vi "HRM-Stage4-init_main.vi"() -> (0 "error out":errorcluster, 3 "Init cluster":T1)   [LabVIEW 2020]
uses:
  HRM-Stage4-init_cluster.ctl
  HRM-Stage4-User_events.ctl
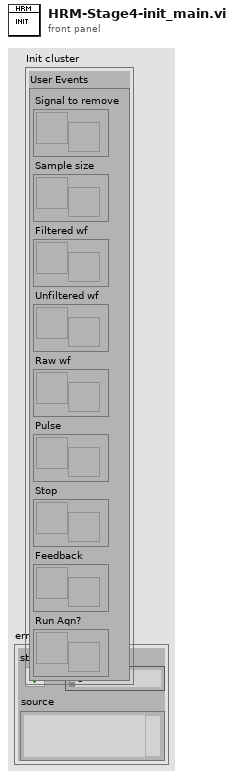
[diagram p1: front panel]
types:
  T1 = typedef "HRM-Stage4-init_cluster.ctl" = cluster{"User Events":T2}
  T2 = typedef "HRM-Stage4-User_events.ctl" = cluster{"Signal to remove":refnum<user-event>, "Sample size":refnum<user-event>, "Filtered wf":refnum<user-event>, "Unfiltered wf":refnum<user-event>, "Raw wf":refnum<user-event>, "Pulse":refnum<user-event>, "Stop":refnum<user-event>, "Feedback":refnum<user-event>, "Run Aqn?":refnum<user-event>}
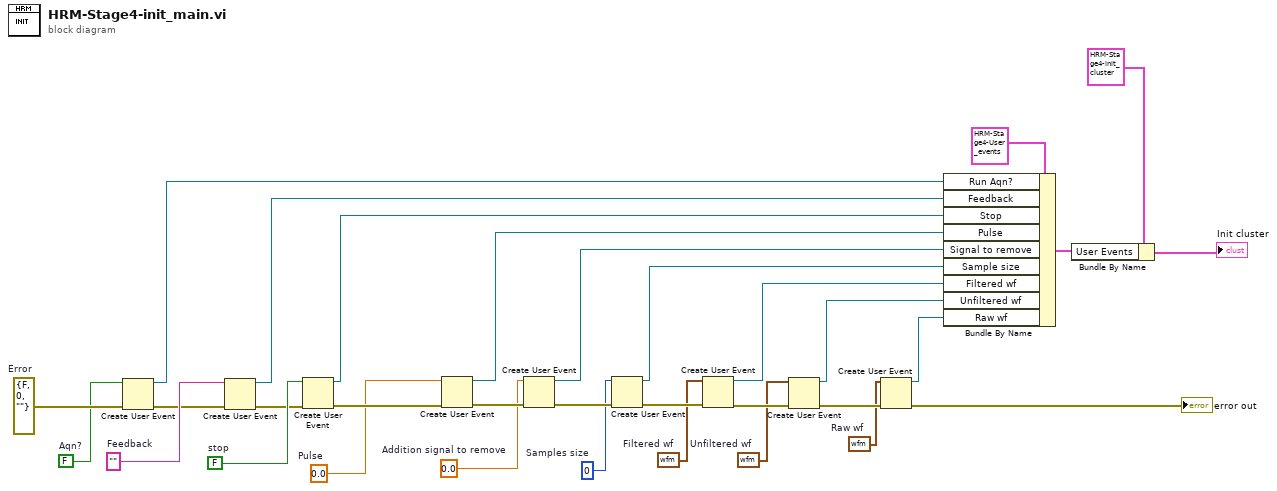
[diagram p0: block diagram]
diagram:
  w2 = FALSE  # Aqn?
  w9 = ""  # Feedback
  w3 = errorcluster {"status"=FALSE, "code"=0, "source"=""}  # Error
  w29 = FALSE  # stop
  w25 = 0.0  # Pulse
  w15 = 0  # Samples size
  w14 = 0.0  # Addition signal to remove
  w13 = waveform(dbl) {"t0"=timestamp(0 s since 1904-01-01), "dt"=1.0, "Y"=[]}  # Filtered wf
  w12 = waveform(dbl) {"t0"=timestamp(0 s since 1904-01-01), "dt"=1.0, "Y"=[]}  # Unfiltered wf
  w11 = waveform(dbl) {"t0"=timestamp(0 s since 1904-01-01), "dt"=1.0, "Y"=[]}  # Raw wf
  n1 = Create User Event(user event datatype=w2, error in=w3) -> (user event=w1:refnum<user-event>, error out=w4:errorcluster)
  n2 = Create User Event(user event datatype=w9, error in=w4) -> (user event=w8:refnum<user-event>, error out=w10:errorcluster)
  n3 = Create User Event(user event datatype=w29, error in=w10) -> (user event=w31:refnum<user-event>, error out=w30:errorcluster)
  n4 = Create User Event(user event datatype=w25, error in=w30) -> (user event=w26:refnum<user-event>, error out=w27:errorcluster)
  n5 = Create User Event(user event datatype=w14, error in=w27) -> (user event=w20:refnum<user-event>, error out=w19:errorcluster)
  n6 = Create User Event(user event datatype=w15, error in=w19) -> (user event=w21:refnum<user-event>, error out=w18:errorcluster)
  n7 = Create User Event(user event datatype=w13, error in=w18) -> (user event=w22:refnum<user-event>, error out=w17:errorcluster)
  n8 = Create User Event(user event datatype=w12, error in=w17) -> (user event=w23:refnum<user-event>, error out=w16:errorcluster)
  n9 = Create User Event(user event datatype=w11, error in=w16) -> (user event=w24:refnum<user-event>, error out=→"error out":errorcluster)
  n10 = Bundle By Name(cluster=T2 {"Signal to remove"=refnum, "Sample size"=refnum, "Filtered wf"=refnum, "Unfiltered wf"=refnum, "Raw wf"=refnum, "Pulse"=refnum, "Stop"=refnum, "Feedback"=refnum, "Run Aqn?"=refnum} ("User Events"), "Run Aqn?"=w1, "Feedback"=w8, "Stop"=w31, "Pulse"=w26, "Signal to remove"=w20, "Sample size"=w21, "Filtered wf"=w22, "Unfiltered wf"=w23, "Raw wf"=w24) -> (w28:T2)
  n11 = Bundle By Name(cluster=T1 {"User Events"={"Signal to remove"=refnum, "Sample size"=refnum, "Filtered wf"=refnum, "Unfiltered wf"=refnum, "Raw wf"=refnum, "Pulse"=refnum, "Stop"=refnum, "Feedback"=refnum, "Run Aqn?"=refnum}} ("Init cluster"), "User Events"=w28) -> (→"Init cluster":T1)
